vi "constants.vi"(8 "error in (no error)":errorcluster, 11 "Small?":bool) -> (0 "error out":errorcluster, 1 "batch updater file path":path, 2 "file path for Signal .hdf5 files":path, 3 "DB connection File Path":path, 4 "file path for Processed Signal .hdf5 files":path, 5 "Testing":bool=TRUE, 6 "Private Folder file path":path)   [LabVIEW 2013]
uses:
  Functional Global Variables/Action Items.ctl
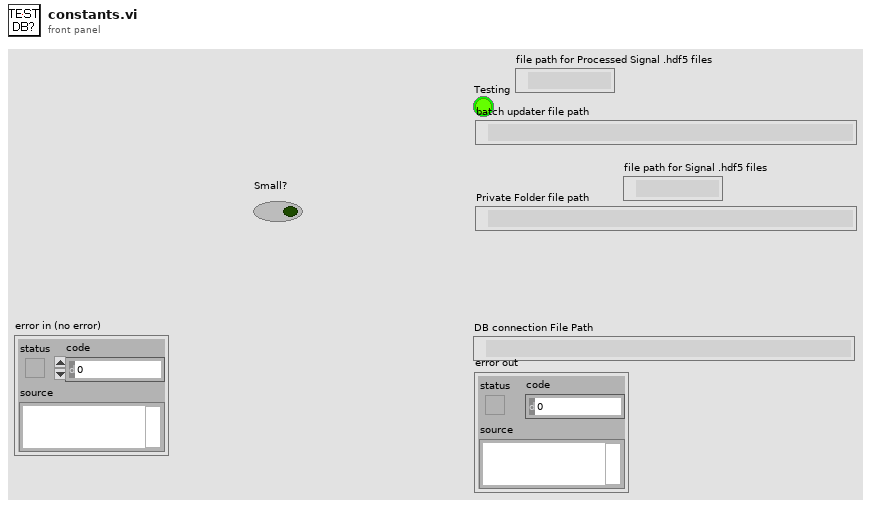
[diagram p1: front panel]
types:
  T1 = typedef "Action Items.ctl" = enum16{"Initialize", "Get", "Set"}
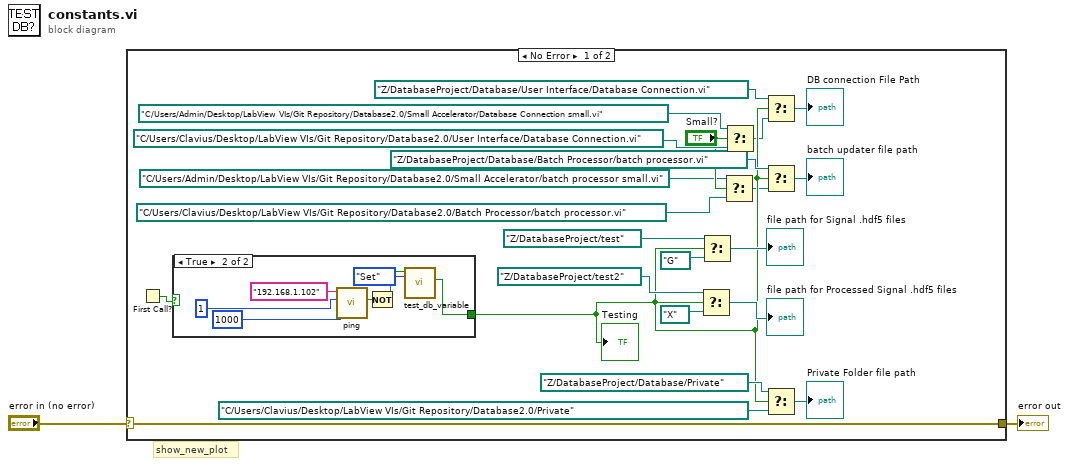
[diagram p0: block diagram]
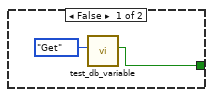
[diagram p2: hidden frame]
diagram:
  # "show_new_plot"
  n1 = case shown="No Error" "error in (no error)" {
    selector: "error in (no error)" -> [w23 w35]
    tunnel: [w23 w35] -> w2
    frame No Error {
      n2 = First Call?() -> (First Call?: T/F=w11:bool)
      n3 = case shown="True" w11 {
        tunnel: [w26 w29] -> w10
        frame False {
          n4 = call "test_db_variable.vi"("Action"=Action_Items."Get") -> ("Test DB out"=w26:bool)  [unwired: 10 in]
        }
        frame True {
          n5 = call "ping.vi"("timeout (ms)"=1000, "count"=1, "host"="192.168.1.102") -> ("found?"=w31:bool)  [unwired: 6 in, 2 out]
          n6 = Not(x=w31) -> (.not. x?=w28:bool)
          n7 = call "test_db_variable.vi"("Action"=Action_Items."Set", "Test DB in"=w28) -> ("Test DB out"=w29:bool)  [unwired: 9 in]
        }
      }
      "Testing" <- w10
      n8 = Select(t=path "Z:/DatabaseProject/test2", s=w10, f=path "X:/") -> (s? t:f=→"file path for Processed Signal .hdf5 files":path)
      n9 = Select(t=path "Z:/DatabaseProject/test", s=w10, f=path "G:/") -> (s? t:f=→"file path for Signal .hdf5 files":path)
      n10 = Select(t=path "C:/Users/Admin/Desktop/LabView VIs/Git Repository/Database2.0/Small Accelerator/batch processor small.vi" ("vi path"), s="Small?", f=path "C:/Users/Clavius/Desktop/LabView VIs/Git Repository/Database2.0/Batch Processor/batch processor.vi" ("vi path")) -> (s? t:f=w5:path)
      n11 = Select(t=path "C:/Users/Admin/Desktop/LabView VIs/Git Repository/Database2.0/Small Accelerator/Database Connection small.vi" ("vi path"), s="Small?", f=path "C:/Users/Clavius/Desktop/LabView VIs/Git Repository/Database2.0/User Interface/Database Connection.vi" ("vi path")) -> (s? t:f=w7:path)
      n12 = Select(t=path "Z:/DatabaseProject/Database/User Interface/Database Connection.vi", s=w10, f=w7) -> (s? t:f=→"DB connection File Path":path)
      n13 = Select(t=path "Z:/DatabaseProject/Database/Batch Processor/batch processor.vi", s=w10, f=w5) -> (s? t:f=→"batch updater file path":path)
      n14 = Select(t=path "Z:/DatabaseProject/Database/Private", s=w10, f=path "C:/Users/Clavius/Desktop/LabView VIs/Git Repository/Database2.0/Private" ("vi path")) -> (s? t:f=→"Private Folder file path":path)
    }
    frame Error {
    }
  }
  "error out" <- w2
